vi "LoadImageListFromXML.vi"(11 "filename":string) -> (3 "Top Sponsor Image List":T1)   [LabVIEW 2013]
uses:
  ImageInfoList.ctl
  <vilib>/Utility/sysdir.llb/System Directory Type.ctl
  <vilib>/Utility/xml.llb/Read From XML File(string).vi
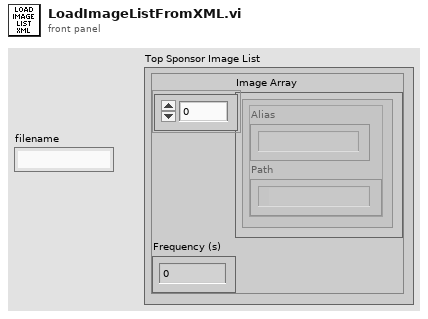
[diagram p1: front panel]
types:
  T1 = typedef "ImageInfoList.ctl" = cluster{"Image Array":cluster{"Alias":string, "Path":path}[], "Frequency (s)":dbl}
  T2 = typedef "System Directory Type.ctl" = i32
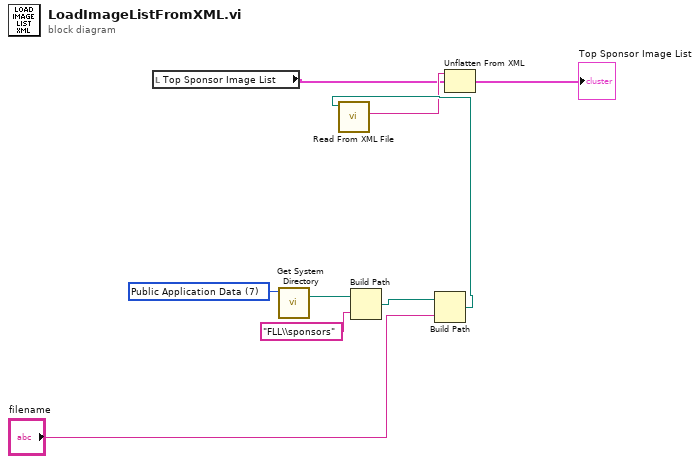
[diagram p0: block diagram]
diagram:
  w6 = T2 7 items=["User Home"=0, "User Desktop"=1, "User Documents"=2, "User Application Data"=3, "User Preferences"=4, "User Temporary"=5, "Public Documents"=6, "Public Application Data"=7, "Public Preferences"=8, "Public Cache"=13, "System Core Libraries"=9, "System Installed Libraries"=10, "Application Files"=11, "Boot Volume Root"=12] ("system directory type")
  n1 = local read "Top Sponsor Image List"() -> (w1:T1)
  n2 = call <vilib>:"Get System Directory.vi"("system directory type"=w6) -> ("system directory"=w4:path)  [unwired: 10 in]
  n3 = Build Path(base path=w4, name or relative path="FLL\\sponsors") -> (appended path=w3:path)
  n4 = Build Path(base path=w3, name or relative path="filename") -> (appended path=w7:path)
  n5 = call-poly <vilib>:"Read From XML File.vi"("XML File Path"=w7) -> ("XML Elements"=w2:string)  [unwired: 8 in, 2 out]
  n6 = Unflatten From XML(xml string=w2, type=w1) -> (value=→"Top Sponsor Image List":T1)  [unwired: 1 in, 1 out]
